vi "TestMode_Local_Read_INI_Sub_VI.vi"(11 "Config File Path":path) -> (2 "output cluster":T1)   [LabVIEW 2017]
uses:
  <vilib>/Utility/config.llb/Read Key (I32).vi
  <vilib>/Utility/config.llb/Read Key (String).vi
  <vilib>/Utility/config.llb/Read Key (Path).vi
  <vilib>/Utility/config.llb/NI_LVConfig.lvlib
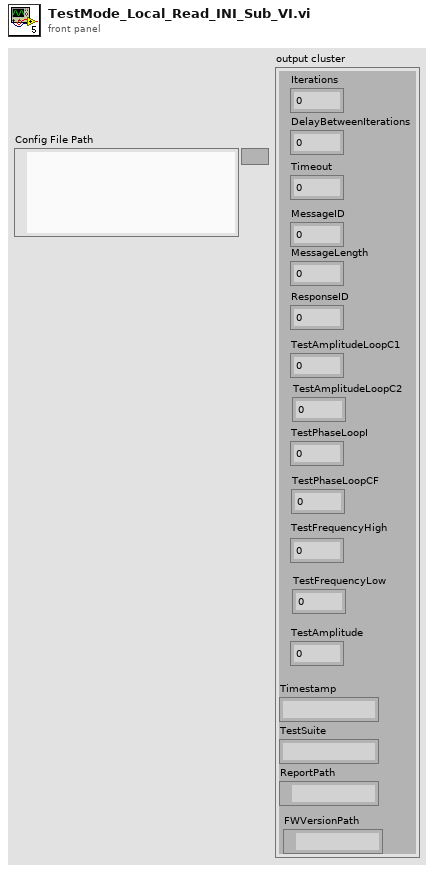
[diagram p1: front panel]
types:
  T1 = cluster{"Iterations":u64, "DelayBetweenIterations":u32, "Timeout":u32, "MessageID":i32, "MessageLength":i32, "ResponseID":i32, "TestAmplitudeLoopC1":i32, "TestAmplitudeLoopC2":i32, "TestPhaseLoopI":i32, "TestPhaseLoopCF":i32, "TestFrequencyHigh":i32, "TestFrequencyLow":i32, "TestAmplitude":i32, "Timestamp":string, "TestSuite":string, "ReportPath":path, "FWVersionPath":path}
  T2 = typedef "NI_LVConfig.lvlib/Config Data RefNum.ctl" = refnum<k1>
  T3 = cluster{u64, u32, u32, i32, i32, i32, i32, i32, i32, i32, i32, i32, i32, "value":string, "value":string, "value":path, path}
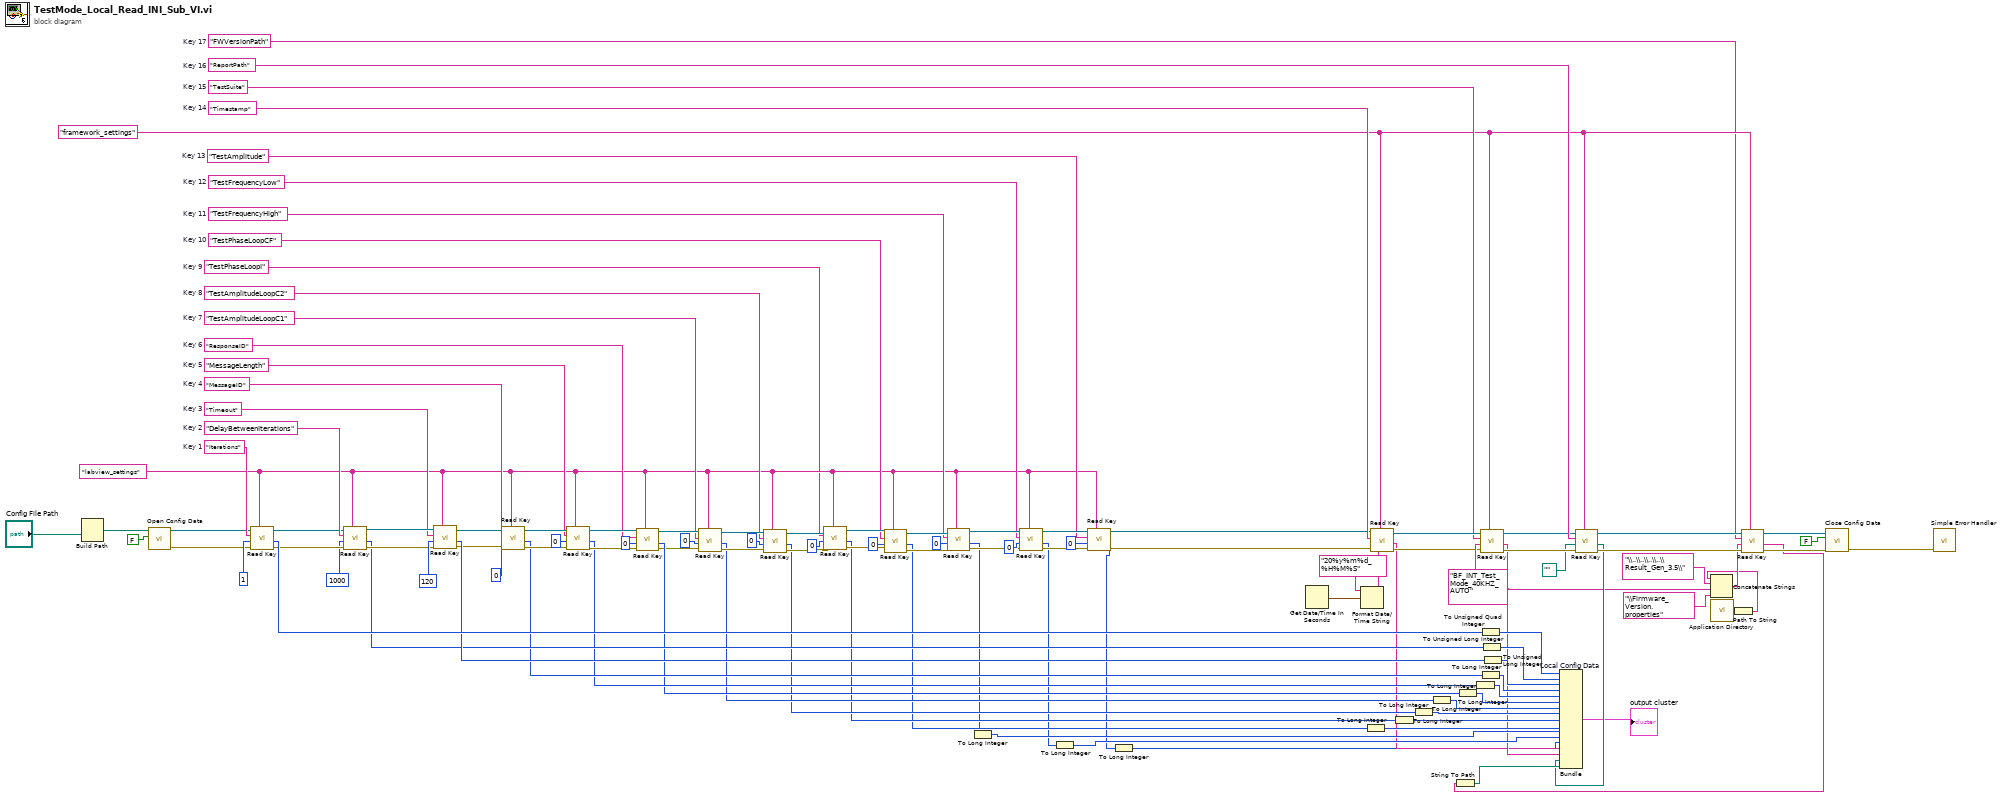
[diagram p0: block diagram]
diagram:
  w9 = "TestAmplitude"  # Key 13
  w38 = "TestFrequencyLow"  # Key 12
  w39 = "TestFrequencyHigh"  # Key 11
  w40 = "TestPhaseLoopCF"  # Key 10
  w4 = "TestPhaseLoopI"  # Key 9
  w41 = "TestAmplitudeLoopC2"  # Key 8
  w42 = "TestAmplitudeLoopC1"  # Key 7
  w58 = "ResponseID"  # Key 6
  w59 = "MessageLength"  # Key 5
  w71 = "MessageID"  # Key 4
  w80 = "FWVersionPath"  # Key 17
  w92 = "Timestamp"  # Key 14
  w87 = "TestSuite"  # Key 15
  w93 = "Timeout"  # Key 3
  w102 = "ReportPath"  # Key 16
  w107 = "DelayBetweenIterations"  # Key 2
  w109 = "Iterations"  # Key 1
  w81 = "framework_settings" ("section")
  w5 = "labview_settings" ("section")
  n1 = Build Path(name or relative path="Config File Path") -> (appended path=w111:path)  [unwired: 1 in]
  n2 = call <vilib>:"Open Config Data.vi"("create file if necessary (T)"=FALSE ("create file if necessary? (T)"), "configuration file path"=w111) -> ("error out"=w74:errorcluster, "refnum"=w73:T2)  [unwired: 7 in, 1 out]
  n3 = call-poly <vilib>:"Read Key.vi"("section"=w5, "error in (no error)"=w74, "default value"=1, "key"=w109, "refnum"=w73) -> ("error out"=w105:errorcluster, "value"=w108:i32, "refnum out"=w106:T2)  [unwired: 4 out]
  n4 = call-poly <vilib>:"Read Key.vi"("section"=w5, "error in (no error)"=w105, "default value"=1000, "key"=w107, "refnum"=w106) -> ("error out"=w100:errorcluster, "value"=w72:i32, "refnum out"=w99:T2)  [unwired: 4 out]
  n5 = call-poly <vilib>:"Read Key.vi"("section"=w5, "error in (no error)"=w100, "default value"=120, "key"=w93, "refnum"=w99) -> ("error out"=w67:errorcluster, "value"=w97:i32, "refnum out"=w70:T2)  [unwired: 4 out]
  n6 = call-poly <vilib>:"Read Key.vi"("section"=w5, "error in (no error)"=w67, "default value"=0, "key"=w71, "refnum"=w70) -> ("error out"=w65:errorcluster, "value"=w64:i32, "refnum out"=w69:T2)  [unwired: 4 out]
  n7 = call-poly <vilib>:"Read Key.vi"("section"=w5, "error in (no error)"=w65, "default value"=0, "key"=w59, "refnum"=w69) -> ("error out"=w66:errorcluster, "value"=w61:i32, "refnum out"=w68:T2)  [unwired: 4 out]
  n8 = call-poly <vilib>:"Read Key.vi"("section"=w5, "error in (no error)"=w66, "default value"=0, "key"=w58, "refnum"=w68) -> ("error out"=w37:errorcluster, "value"=w60:i32, "refnum out"=w48:T2)  [unwired: 4 out]
  n9 = call-poly <vilib>:"Read Key.vi"("section"=w5, "error in (no error)"=w37, "default value"=0, "key"=w42, "refnum"=w48) -> ("error out"=w33:errorcluster, "value"=w28:i32, "refnum out"=w47:T2)  [unwired: 4 out]
  n10 = call-poly <vilib>:"Read Key.vi"("section"=w5, "error in (no error)"=w33, "default value"=0, "key"=w41, "refnum"=w47) -> ("error out"=w36:errorcluster, "value"=w26:i32, "refnum out"=w46:T2)  [unwired: 4 out]
  n11 = call-poly <vilib>:"Read Key.vi"("section"=w5, "error in (no error)"=w36, "default value"=0, "key"=w4, "refnum"=w46) -> ("error out"=w35:errorcluster, "value"=w24:i32, "refnum out"=w45:T2)  [unwired: 4 out]
  n12 = call-poly <vilib>:"Read Key.vi"("section"=w5, "error in (no error)"=w35, "default value"=0, "key"=w40, "refnum"=w45) -> ("error out"=w32:errorcluster, "value"=w22:i32, "refnum out"=w44:T2)  [unwired: 4 out]
  n13 = call-poly <vilib>:"Read Key.vi"("section"=w5, "error in (no error)"=w32, "default value"=0, "key"=w39, "refnum"=w44) -> ("error out"=w34:errorcluster, "value"=w20:i32, "refnum out"=w43:T2)  [unwired: 4 out]
  n14 = To Long Integer(number=w20) -> (32bit integer=w19:i32)
  n15 = call-poly <vilib>:"Read Key.vi"("section"=w5, "error in (no error)"=w34, "default value"=0, "key"=w38, "refnum"=w43) -> ("error out"=w17:errorcluster, "value"=w16:i32, "refnum out"=w15:T2)  [unwired: 4 out]
  n16 = To Long Integer(number=w16) -> (32bit integer=w18:i32)
  n17 = call-poly <vilib>:"Read Key.vi"("section"=w5, "error in (no error)"=w17, "default value"=0, "key"=w9, "refnum"=w15) -> ("error out"=w2:errorcluster, "value"=w7:i32, "refnum out"=w3:T2)  [unwired: 4 out]
  n18 = To Long Integer(number=w7) -> (32bit integer=w6:i32)
  n19 = Get Date/Time In Seconds() -> (seconds since 1Jan1904=w94:timestamp)
  n20 = Format Date/Time String(time format string (%c)="20%y%m%d_%H%M%S", seconds (now)=w94) -> (date/time string=w95:string)  [unwired: 1 out]
  n21 = To Long Integer(number=w22) -> (32bit integer=w21:i32)
  n22 = call-poly <vilib>:"Read Key.vi"("section"=w81, "error in (no error)"=w2, "default value"=w95, "key"=w92, "refnum"=w3) -> ("error out"=w89:errorcluster, "value"=w10:string, "refnum out"=w90:T2)  [unwired: 1 in, 3 out]
  n23 = To Long Integer(number=w24) -> (32bit integer=w23:i32)
  n24 = To Long Integer(number=w26) -> (32bit integer=w25:i32)
  n25 = To Long Integer(number=w28) -> (32bit integer=w27:i32)
  n26 = To Long Integer(number=w60) -> (32bit integer=w31:i32)
  n27 = To Long Integer(number=w61) -> (32bit integer=w62:i32)
  n28 = To Unsigned Quad Integer(1:w108) -> (0:w115:u64)
  n29 = To Long Integer(number=w64) -> (32bit integer=w63:i32)
  n30 = call-poly <vilib>:"Read Key.vi"("section"=w81, "error in (no error)"=w89, "default value"="BF_INT_Test_Mode_40KHZ_AUTO", "key"=w87, "refnum"=w90) -> ("error out"=w88:errorcluster, "value"=w11:string, "refnum out"=w91:T2)  [unwired: 1 in, 3 out]
  n31 = To Unsigned Long Integer(number=w72) -> (unsigned 32bit integer=w30:u32)
  n32 = To Unsigned Long Integer(number=w97) -> (unsigned 32bit integer=w29:u32)
  n33 = call-poly <vilib>:"Read Key.vi"("section"=w81, "error in (no error)"=w88, "default value"=path "", "key"=w102, "refnum"=w91) -> ("error out"=w82:errorcluster, "value"=w12:path, "refnum out"=w85:T2)  [unwired: 1 in, 3 out]
  n34 = call <vilib>:"Application Directory.vi"() -> ("Application Directory"=w76:path)
  n35 = Path To String(path=w76) -> (string=w75:string)
  n36 = Concatenate Strings(w75, "\\..\\..\\..\\..\\Result_Gen_3.5\\" ("default value"), w11, "\\Firmware_Version.properties" ("default value")) -> (w79:string)
  n37 = call-poly <vilib>:"Read Key.vi"("section"=w81, "error in (no error)"=w82, "default value"=w79, "key"=w80, "refnum"=w85) -> ("error out"=w83:errorcluster, "value"=w14:string, "refnum out"=w84:T2)  [unwired: 1 in, 3 out]
  n38 = String To Path(string=w14) -> (path=w13:path)
  n39 = Bundle "Local Config Data"(w115, w30, w29, w63, w62, w31, w27, w25, w23, w21, w19, w18, w6, "value"=w10, "value"=w11, "value"=w12, w13) -> (→"output cluster":T3)  [unwired: 1 in]
  n40 = call <vilib>:"Close Config Data.vi"("error in (no error)"=w83, "write file if changed (T)"=FALSE ("write configuration file? (T)"), "refnum"=w84) -> ("error out"=w112:errorcluster)  [unwired: 8 out]
  n41 = call <vilib>:"Simple Error Handler.vi"("error in (no error)"=w112) -> ()  [unwired: 1 in, 8 out]
